vi "Do Something Else.vi"(8 "error in (no error)":errorcluster, 9 "X":dbl, 10 "Do Something Message":string, 11 "TemplateAPI in":refnum<class "ExampleAPI.lvclass">) -> (0 "error out":errorcluster, 3 "TemplateAPI out":refnum<class "ExampleAPI.lvclass">)   [LabVIEW 2018, in "ExampleAPI.lvclass"]
uses:
  ExampleAPI.lvclass
  C:/Users/Phalanx/Documents/LabVIEW-Application-API-Template/src/Classes/AppControlAPI/AppControlAPI.lvclass
  AppControlAPI/AppControlAPI.lvclass/AppControlAPI.ctl
  4c94efee-2ba9-4b86-bf77-9303cd5a5534.vi
  AppControlAPI/Read AppRef.vi
  AppControlAPI/Insert In Reference Cache.vi
  AppControlAPI/Read Cache.vi
  AppControlAPI/Write Cache.vi
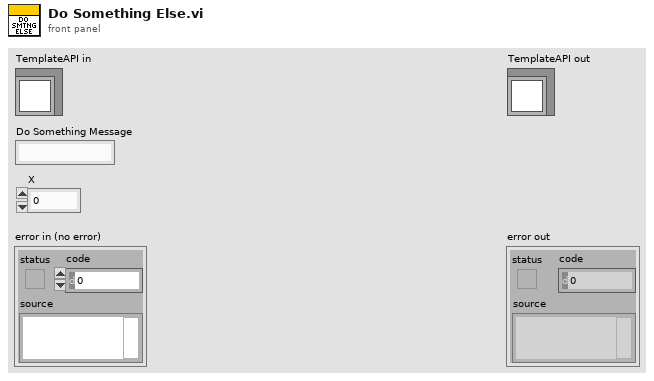
[diagram p1: front panel]
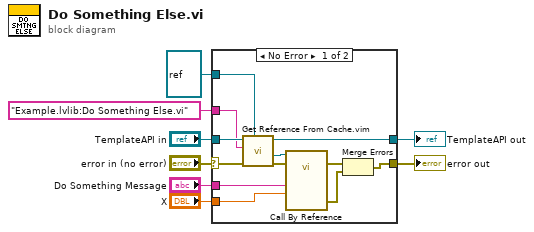
[diagram p0: block diagram]
diagram:
  n1 = case shown="No Error" "error in (no error)" {
    selector: "error in (no error)" -> [w16 w22]
    tunnel: [w13 w22] -> w7
    tunnel: [w19 w21] -> w5
    tunnel: "TemplateAPI in" -> [w20 w21]
    tunnel: "Do Something Message" -> [w14 _]
    tunnel: "Example.lvlib:Do Something Else.vi" ("VIQualifiedName") -> [w11 _]
    tunnel: refnum<vi> refnum ("type specifier VI Refnum (for type only)") -> [w10 _]
    tunnel: "X" -> [w9 _]
    frame No Error {
      n2 = call "Get Reference From Cache.vim"("type specifier VI Refnum (for type only)"=w10, "error in (no error)"=w16, "VIQualifiedName"=w11, "AppControlAPI in"=w20) -> ("error out"=w17:errorcluster, "VIRef"=w18:refnum<vi>, "AppControlAPI out"=w19:refnum<class "ExampleAPI.lvclass">)  [unwired: 5 in]
      n3 = call-by-ref "?"(reference=w18, error in=w17, "X"=w9, "Do Something Else Message"=w14) -> (error out=w15:errorcluster, 0:"error out"=w12:errorcluster)  [unwired: 9 in, 1 out]
      n4 = Merge Errors(w15, w12) -> (w13:errorcluster)
    }
    frame Error {
    }
  }
  "error out" <- w7
  "TemplateAPI out" <- w5
